vi "FPGA_ZApproachStep.vi"() -> ()   [LabVIEW 2014]
uses:
  <vilib>/rvi/Emulation/niFpgaGetClockAttributes.vi
  <vilib>/rvi/Emulation/niFpgaSctlEmulationGetInTimedLoop.vi
  <vilib>/rvi/Emulation/niFpgaEmulationReportErrorSimple.vi
  <vilib>/rvi/eio/common/nirviEmuTemplateMethod_errors.vi
  <vilib>/rvi/Emulation/niFpgaCriticalErrorInLSC.vi
  <vilib>/rvi/Emulation/niFpgaProcessEmulError.vi
  <vilib>/eio/EIONode/EIONode.xnode
panel:
  out "PresCurr":i16
  out "CalPIZPos":i16
  out "RealPIZPos":i16
  in  "stop":bool
  out "OverUppedLimit?":bool
  out "Approached?":bool
  out "RangeExceeded?":bool
  in  "RefCurr":i16
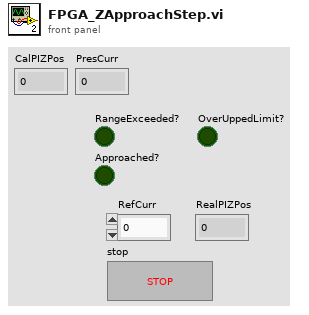
[diagram p1: front panel]
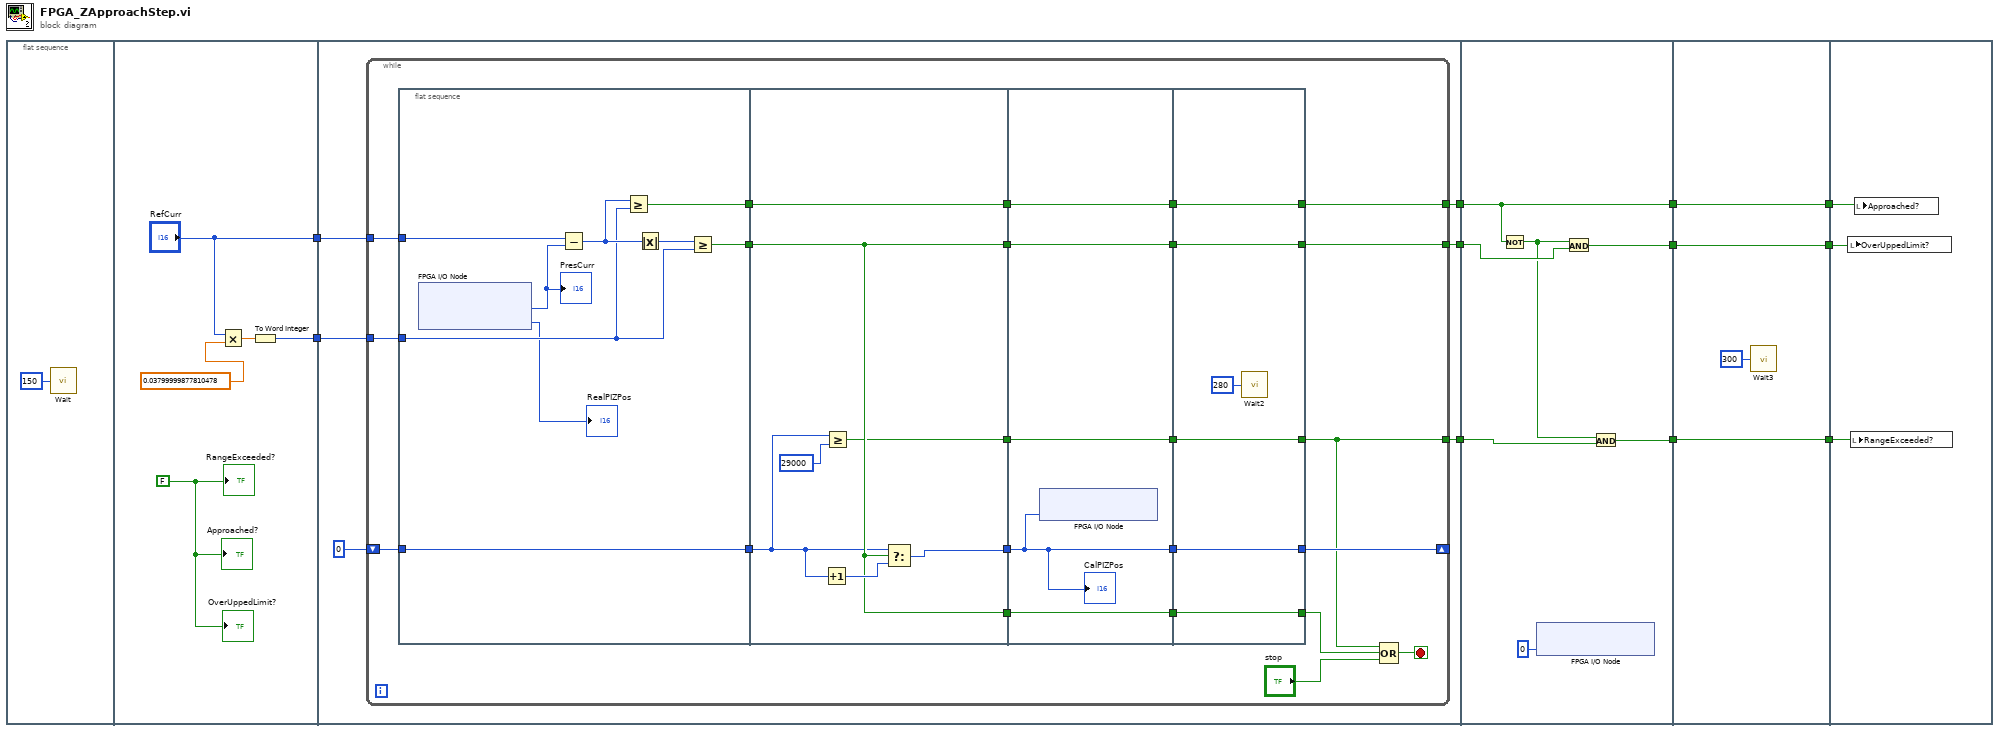
[diagram p0: block diagram]
diagram:
  n1 = flat-sequence {
    tunnel: [w14] -> w11
    tunnel: ["RefCurr"] -> w10
    tunnel: w11 -> [w22]
    tunnel: w10 -> [w23]
    tunnel: [w20] -> w9
    tunnel: [w19] -> w8
    tunnel: [w18] -> w7
    tunnel: w9 -> [w78]
    tunnel: w8 -> [w79]
    tunnel: w7 -> [w74]
    tunnel: [w78] -> w6
    tunnel: [w76] -> w4
    tunnel: [w77] -> w2
    tunnel: w6 -> [w83]
    tunnel: [w83] -> w5
    tunnel: w4 -> [w82]
    tunnel: [w82] -> w3
    tunnel: w2 -> [w81]
    tunnel: [w81] -> w1
    tunnel: w5 -> [w87]
    tunnel: w3 -> [w85]
    tunnel: w1 -> [w86]
    frame #0 {
      n2 = call "Wait"("Count(mSec)"=u32 150) -> ()  [unwired: 1 out]
    }
    frame #1 {
      w17 = FALSE
      n3 = Multiply(x="RefCurr", y=sgl 0.038) -> (x*y=w15:sgl)
      n4 = To Word Integer(number=w15) -> (16bit integer=w14:i16)
      "RangeExceeded?" <- w17
      "Approached?" <- w17
      "OverUppedLimit?" <- w17
    }
    frame #2 {
      n5 = while {
        tunnel: w23 -> [w46]
        tunnel: w22 -> [w45]
        shift-right: [w40] -> _
        shift-left: i16 0 -> [w44]
        tunnel: [w28] -> w20
        tunnel: [w27] -> w19
        tunnel: [w24] -> w18
        stop <- w33 stop-if-true
        n6 = flat-sequence {
          tunnel: w46 -> [w55]
          tunnel: w45 -> [w51]
          tunnel: w44 -> [w50]
          tunnel: [w50] -> w43
          tunnel: [w49] -> w39
          tunnel: [w48] -> w38
          tunnel: w43 -> [w58]
          tunnel: [w62] -> w41
          tunnel: w39 -> [w59]
          tunnel: w38 -> [w60]
          tunnel: [w60] -> w37
          tunnel: [w59] -> w36
          tunnel: [w59] -> w31
          tunnel: [w56] -> w26
          tunnel: [w67] -> w42
          tunnel: w41 -> [w67]
          tunnel: w37 -> [w64]
          tunnel: w36 -> [w66]
          tunnel: [w66] -> w35
          tunnel: w31 -> [w65]
          tunnel: [w65] -> w30
          tunnel: [w64] -> w29
          tunnel: w26 -> [w63]
          tunnel: [w63] -> w25
          tunnel: w42 -> [w73]
          tunnel: [w73] -> w40
          tunnel: w35 -> [w72]
          tunnel: [w72] -> w32
          tunnel: w30 -> [w71]
          tunnel: [w71] -> w27
          tunnel: [w70] -> w28
          tunnel: w29 -> [w70]
          tunnel: [w68] -> w24
          tunnel: w25 -> [w68]
          frame #0 {
            n7 = xnode "FPGA I/O Node"() -> ("Connector0/AI1"=w54:i16, "Connector0/AI0"=→"RealPIZPos":i16)  [unwired: 2 in, 2 out]
            "PresCurr" <- w54
            n8 = Subtract(x=w55, y=w54) -> (x-y=w52:i16)
            n9 = Greater Or Equal?(x=w52, y=w51) -> (x >= y?=w48:bool)
            n10 = Absolute Value(x=w52) -> (abs(x)=w53:i16)
            n11 = Greater Or Equal?(x=w53, y=w51) -> (x >= y?=w49:bool)
          }
          frame #1 {
            n12 = Increment(x=w58) -> (x+1=w61:i16)
            n13 = Greater Or Equal?(x=w58, y=i16 29000) -> (x >= y?=w56:bool)
            n14 = Select(t=w58, s=w59, f=w61) -> (s? t:f=w62:i16)
          }
          frame #2 {
            n15 = xnode "FPGA I/O Node"("Connector0/AO0"=w67) -> ()  [unwired: 1 in, 1 out]
            "CalPIZPos" <- w67
          }
          frame #3 {
            n16 = call "Wait2"("Count(uSec)"=u32 280) -> ()  [unwired: 1 out]
          }
        }
        n17 = Compound Arithmetic op=OR(w24, w32, "stop") -> (w33:bool)
      }
    }
    frame #3 {
      n18 = Not(x=w78) -> (.not. x?=w75:bool)
      n19 = xnode "FPGA I/O Node"("Connector0/AO0"=i16 0) -> ()  [unwired: 1 in, 1 out]
      n20 = And(x=w75, y=w79) -> (x .and. y?=w77:bool)
      n21 = And(x=w75, y=w74) -> (x .and. y?=w76:bool)
    }
    frame #4 {
      n22 = call "Wait3"("Count(uSec)"=u32 300) -> ()  [unwired: 1 out]
    }
    frame #5 {
      n23 = local write "OverUppedLimit?"(w86) -> ()
      n24 = local write "RangeExceeded?"(w85) -> ()
      n25 = local write "Approached?"(w87) -> ()
    }
  }
